vi "FtoT.vi"(4 "DesiredFM":dbl[](array[numeric]), 7 "cables unit vect":T1) -> (1 "desiredT":dbl[](array[numeric]))   [LabVIEW 2017]
uses:
  <vilib>/Analysis/Matrix/Datatypes/RealMatrix.ctl
  <vilib>/Analysis/baseanly.llb/Real Dot Product.vi
  <vilib>/Analysis/NI_AALBase.lvlib
  <vilib>/Analysis/Matrix/NI_Matrix.lvlib
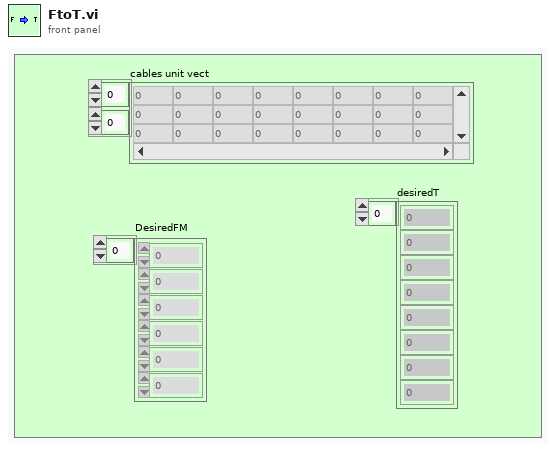
[diagram p1: front panel]
types:
  T1 = typedef "NI_Matrix.lvlib/RealMatrix.ctl" = dbl[][]
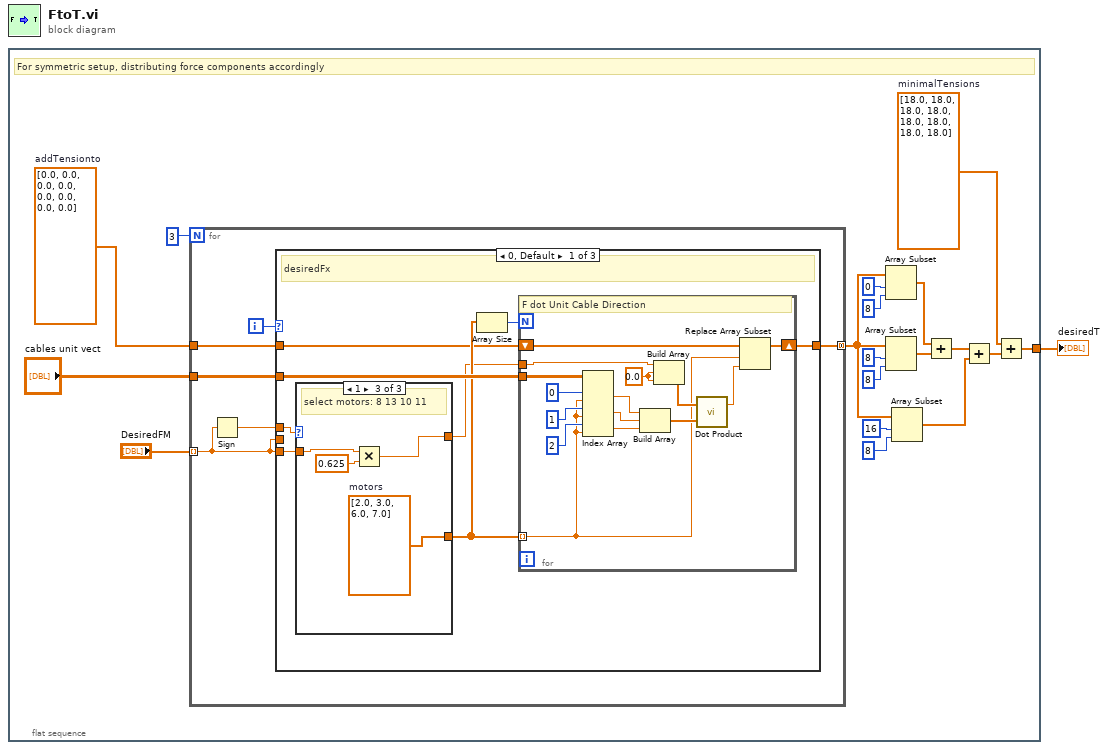
[diagram p0: block diagram]
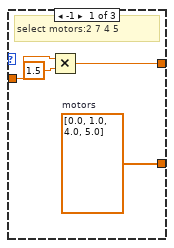
[diagram p2: hidden frame]
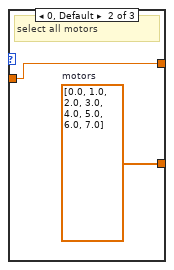
[diagram p3: hidden frame]
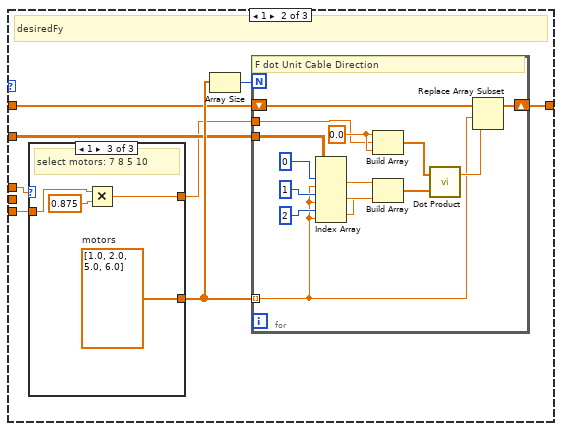
[diagram p4: hidden frame]
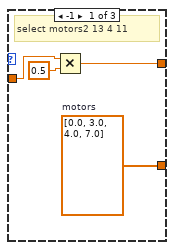
[diagram p5: hidden frame]
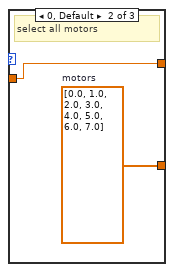
[diagram p6: hidden frame]
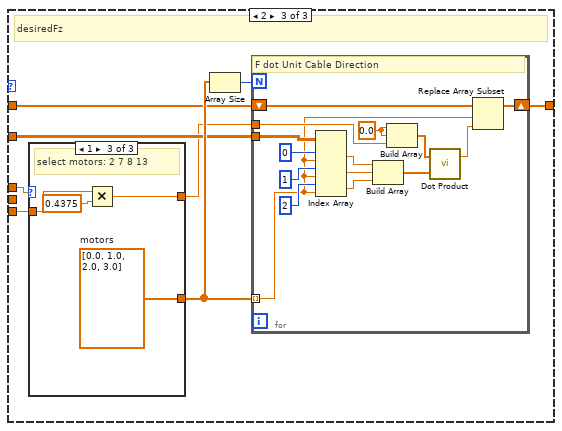
[diagram p7: hidden frame]
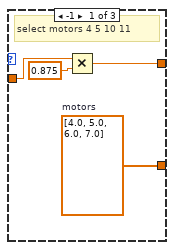
[diagram p8: hidden frame]
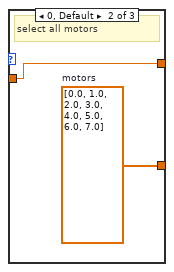
[diagram p9: hidden frame]
diagram:
  n1 = flat-sequence {
    tunnel: [w15] -> w1
    frame #0 {
      w14 = dbl[] [0.0, 0.0, 0.0, 0.0, 0.0, 0.0, 0.0, 0.0]  # addTensionto
      w16 = dbl[] [18.0, 18.0, 18.0, 18.0, 18.0, 18.0, 18.0, 18.0]  # minimalTensions
      # "For symmetric setup, distributing force components accordingly"
      n2 = for {
        N: 3 -> [_]
        tunnel: "DesiredFM" -> [w20] mode=indexing
        tunnel: "cables unit vect" -> [w23]
        tunnel: w14 -> [w22]
        tunnel: [w21] -> w4 mode=concatenating
        i -> [w25]
        n3 = Sign(1:w20) -> (0:w24:dbl)
        n4 = case shown="0, Default" w25 {
          tunnel: w24 -> [w33 w63 w96]
          tunnel: w23 -> [w32 w64 w97]
          tunnel: w20 -> [_ _ _]
          tunnel: w22 -> [w29 w62 w95]
          tunnel: [w28 w61 w94] -> w21
          tunnel: w20 -> [w27 w60 w93]
          frame 0, Default {
            # "desiredFx"
            n5 = case shown="1" w33 {
              tunnel: [w52 w54 w58] -> w31
              tunnel: w27 -> [w51 w53 w57]
              tunnel: [w49 w53 w55] -> w26
              frame -1 {
                w52 = dbl[] [0.0, 1.0, 4.0, 5.0]  # motors
                # "select motors:2 7 4 5"
                n6 = Multiply(x=w51, y=1.5) -> (x*y=w49:dbl)
              }
              frame 0, Default {
                w54 = dbl[] [0.0, 1.0, 2.0, 3.0, 4.0, 5.0, 6.0, 7.0]  # motors
                # "select all motors"
              }
              frame 1 {
                w58 = dbl[] [2.0, 3.0, 6.0, 7.0]  # motors
                # "select motors: 8 13 10 11"
                n7 = Multiply(x=w57, y=0.625) -> (x*y=w55:dbl)
              }
            }
            n8 = Array Size(array=w31) -> (size(s)=w30:i32)
            n9 = for {
              N: w30 -> [_]
              tunnel: w32 -> [w48]
              tunnel: w31 -> [w37] mode=indexing
              tunnel: w26 -> [w40]
              shift-right: [w35] -> w28
              shift-left: w29 -> [w34]
              w39 = 0.0 ("element")
              # "F dot Unit Cable Direction"
              n10 = Index Array(array=w48, index (row) #1=0 ("index (row)"), index (col) #1=w37, index (row) #2=1 ("index (row)"), index (col) #2=w37, index (row) #3=2 ("index (row)"), index (col) #3=w37) -> (element #1=w44:dbl, element #2=w43:dbl, element #3=w42:dbl)
              n11 = Build Array(w44, w43, w42) -> (w41:dbl[])
              n12 = Build Array(w40, w39, w39) -> (w38:dbl[])
              n13 = call-poly <vilib>:"Dot Product.vi"("Y Vector"=w41, "X Vector"=w38) -> ("X * Y"=w36:dbl)  [unwired: 1 out]
              n14 = Replace Array Subset(array=w34, new element=w36, index=w37) -> (w35:dbl[])
            }
          }
          frame 1 {
            # "desiredFy"
            n15 = case shown="1" w63 {
              tunnel: [w85 w87 w91] -> w66
              tunnel: w60 -> [w84 w86 w90]
              tunnel: [w82 w86 w88] -> w59
              frame -1 {
                w85 = dbl[] [0.0, 3.0, 4.0, 7.0]  # motors
                # "select motors2 13 4 11"
                n16 = Multiply(x=w84, y=0.5) -> (x*y=w82:dbl)
              }
              frame 0, Default {
                w87 = dbl[] [0.0, 1.0, 2.0, 3.0, 4.0, 5.0, 6.0, 7.0]  # motors
                # "select all motors"
              }
              frame 1 {
                w91 = dbl[] [1.0, 2.0, 5.0, 6.0]  # motors
                # "select motors: 7 8 5 10"
                n17 = Multiply(x=w90, y=0.875) -> (x*y=w88:dbl)
              }
            }
            n18 = Array Size(array=w66) -> (size(s)=w65:i32)
            n19 = for {
              N: w65 -> [_]
              tunnel: w64 -> [w81]
              tunnel: w66 -> [w70] mode=indexing
              shift-right: [w68] -> w61
              shift-left: w62 -> [w69]
              tunnel: w59 -> [w67]
              w72 = 0.0 ("element")
              # "F dot Unit Cable Direction"
              n20 = Index Array(array=w81, index (row) #1=0 ("index (row)"), index (col) #1=w70, index (row) #2=1 ("index (row)"), index (col) #2=w70, index (row) #3=2 ("index (row)"), index (col) #3=w70) -> (element #1=w77:dbl, element #2=w76:dbl, element #3=w75:dbl)
              n21 = Build Array(w72, w67, w72) -> (w73:dbl[])
              n22 = Build Array(w77, w76, w75) -> (w74:dbl[])
              n23 = call-poly <vilib>:"Dot Product.vi"("Y Vector"=w74, "X Vector"=w73) -> ("X * Y"=w71:dbl)  [unwired: 1 out]
              n24 = Replace Array Subset(array=w69, new element=w71, index=w70) -> (w68:dbl[])
            }
          }
          frame 2 {
            # "desiredFz"
            n25 = case shown="1" w96 {
              tunnel: [w118 w120 w124] -> w99
              tunnel: w93 -> [w117 w119 w123]
              tunnel: [w115 w119 w121] -> w92
              frame -1 {
                w118 = dbl[] [4.0, 5.0, 6.0, 7.0]  # motors
                # "select motors 4 5 10 11"
                n26 = Multiply(x=w117, y=0.875) -> (x*y=w115:dbl)
              }
              frame 0, Default {
                w120 = dbl[] [0.0, 1.0, 2.0, 3.0, 4.0, 5.0, 6.0, 7.0]  # motors
                # "select all motors"
              }
              frame 1 {
                w124 = dbl[] [0.0, 1.0, 2.0, 3.0]  # motors
                # "select motors: 2 7 8 13"
                n27 = Multiply(x=w123, y=0.4375) -> (x*y=w121:dbl)
              }
            }
            n28 = Array Size(array=w99) -> (size(s)=w98:i32)
            n29 = for {
              N: w98 -> [_]
              tunnel: w97 -> [w114]
              tunnel: w99 -> [w100] mode=indexing
              tunnel: w92 -> [w104]
              shift-right: [w101] -> w94
              shift-left: w95 -> [w102]
              w105 = 0.0 ("element")
              # "F dot Unit Cable Direction"
              n30 = Index Array(array=w114, index (row) #1=0 ("index (row)"), index (col) #1=w100, index (row) #2=1 ("index (row)"), index (col) #2=w100, index (row) #3=2 ("index (row)"), index (col) #3=w100) -> (element #1=w110:dbl, element #2=w109:dbl, element #3=w108:dbl)
              n31 = Build Array(w110, w109, w108) -> (w107:dbl[])
              n32 = Build Array(w105, w105, w104) -> (w106:dbl[])
              n33 = call-poly <vilib>:"Dot Product.vi"("Y Vector"=w107, "X Vector"=w106) -> ("X * Y"=w103:dbl)  [unwired: 1 out]
              n34 = Replace Array Subset(array=w102, new element=w103, index=w100) -> (w101:dbl[])
            }
          }
        }
      }
      n35 = Array Subset(array=w4, index=0, length=8) -> (w11:dbl[])
      n36 = Array Subset(array=w4, index=8, length=8) -> (w8:dbl[])
      n37 = Array Subset(array=w4, index=16, length=8) -> (w3:dbl[])
      n38 = Add(x=w11, y=w8) -> (x+y=w7:dbl[])
      n39 = Add(x=w7, y=w3) -> (x+y=w2:dbl[])
      n40 = Add(x=w16, y=w2) -> (x+y=w15:dbl[])
    }
  }
  "desiredT" <- w1
